vi "IP键盘.vi"(1 "OldNumber":string) -> (0 "NewNumber":string)   [LabVIEW 2016, in "数据传输系统-05.lvlib"]
panel:
  in  "数值":dbl
  in  "Cancel":bool
  in  "OK":bool
  in  "Clear":bool
  in  "BackSpace":bool
  in  "String":string
  in  "Point":bool
  in  "Zero":bool
  in  "Nine":bool
  in  "Eight":bool
  in  "Seven":bool
  in  "Six":bool
  in  "Five":bool
  in  "Four":bool
  in  "Three":bool
  in  "Two":bool
  in  "One":bool
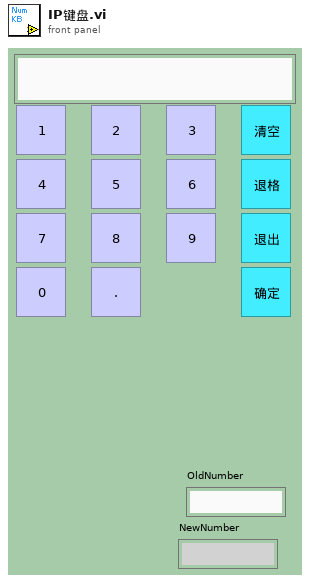
[diagram p1: front panel]
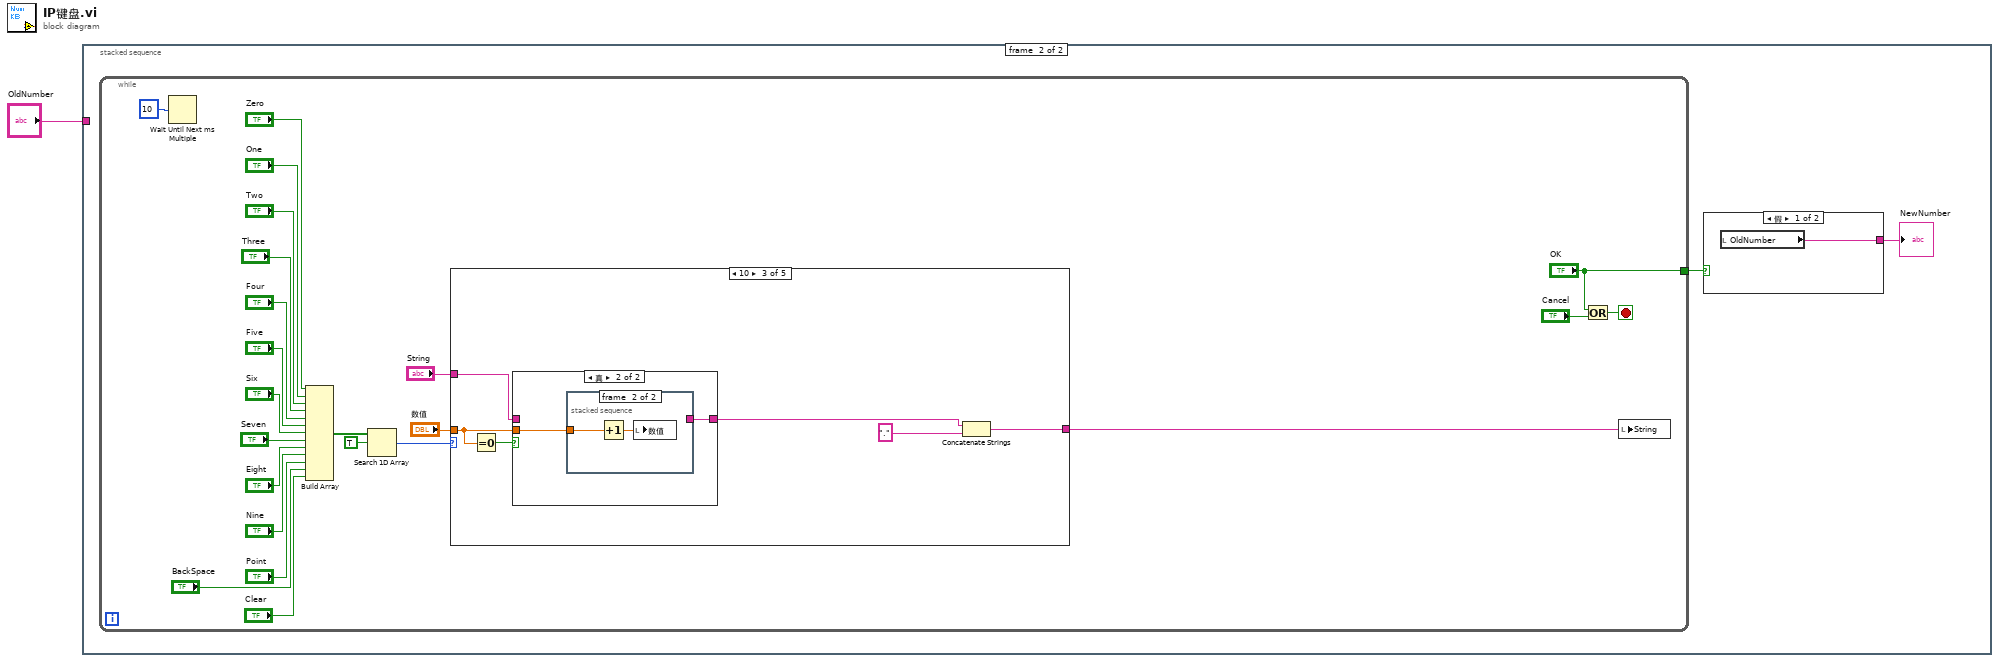
[diagram p0: block diagram]
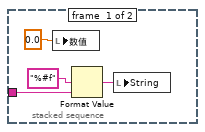
[diagram p2: hidden frame]
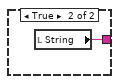
[diagram p3: hidden frame]
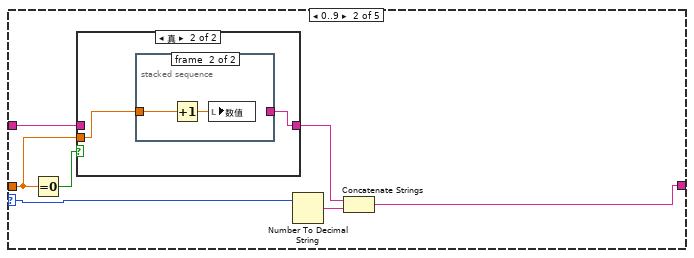
[diagram p5: hidden frame]
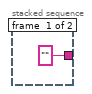
[diagram p7: hidden frame]
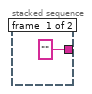
[diagram p9: hidden frame]
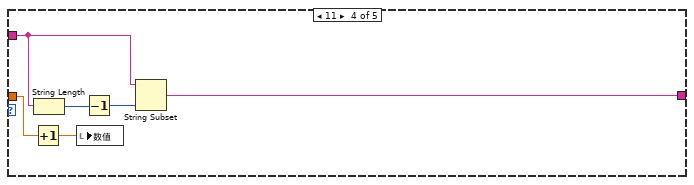
[diagram p10: hidden frame]
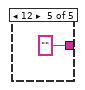
[diagram p11: hidden frame]
diagram:
  n1 = stacked-sequence {
    tunnel: "OldNumber" -> [w2 _]
    frame #0 {
      n2 = local write "数值"(0.0 ("数值")) -> ()
      n3 = Format Value(format string="%#f" ("格式字符串"), value (0)=w2) -> (output string=w3:string)  [unwired: 1 in]
      n4 = local write "String"(w3) -> ()
    }
    frame #1 {
      n5 = while {
        tunnel: ["OK"] -> w7
        stop <- w31 stop-if-true
        n6 = Wait Until Next ms Multiple(millisecond multiple=u32 10) -> ()  [unwired: 1 out]
        n7 = Build Array("Zero", "One", "Two", "Three", "Four", "Five", "Six", "Seven", "Eight", "Nine", "Point", "BackSpace", "Clear") -> (w16:bool[])
        n8 = Search 1D Array(1D array=w16, element=TRUE) -> (index of element=w14:i32)  [unwired: 1 in]
        n9 = case shown="10" w14 {
          selector: w14 -> [_ w40 _ _ _]
          tunnel: "String" -> [w33 w35 w51 w63 _]
          tunnel: [w33 w38 w52 w61 "" ("String")] -> w10
          tunnel: "数值" -> [_ w34 w48 w60 _]
          frame Default {
          }
          frame 0..9 {
            n10 = Equal To 0?(x=w34) -> (x = 0?=w37:bool)
            n11 = case shown="真" w37 {
              tunnel: [w41 w43] -> w36
              tunnel: w34 -> [_ w42]
              tunnel: w35 -> [w41 _]
              frame False {
              }
              frame True {
                n12 = stacked-sequence {
                  tunnel: ["" _] -> w43
                  tunnel: w42 -> [_ w46]
                  frame #0 {
                  }
                  frame #1 {
                    n13 = Increment(x=w46) -> (x+1=w45:dbl)
                    n14 = local write "数值"(w45) -> ()
                  }
                }
              }
            }
            n15 = Number To Decimal String(number=w40) -> (decimal integer string=w39:string)  [unwired: 1 in]
            n16 = Concatenate Strings(w36, w39) -> (w38:string)
          }
          frame 10 {
            n17 = Equal To 0?(x=w48) -> (x = 0?=w50:bool)
            n18 = case shown="真" w50 {
              tunnel: [w53 w55] -> w49
              tunnel: w51 -> [w53 _]
              tunnel: w48 -> [_ w54]
              frame False {
              }
              frame True {
                n19 = stacked-sequence {
                  tunnel: ["" _] -> w55
                  tunnel: w54 -> [_ w57]
                  frame #0 {
                  }
                  frame #1 {
                    n20 = Increment(x=w57) -> (x+1=w58:dbl)
                    n21 = local write "数值"(w58) -> ()
                  }
                }
              }
            }
            n22 = Concatenate Strings(w49, "." ("string")) -> (w52:string)
          }
          frame 11 {
            n23 = Increment(x=w60) -> (x+1=w59:dbl)
            n24 = String Length(string=w63) -> (length=w62:i32)
            n25 = local write "数值"(w59) -> ()
            n26 = Decrement(x=w62) -> (x-1=w64:i32)
            n27 = String Subset(string=w63, length (rest)=w64) -> (substring=w61:string)  [unwired: 1 in]
          }
          frame 12 {
          }
        }
        n28 = Or(x="OK", y="Cancel") -> (x .or. y?=w31:bool)
        n29 = local write "String"(w10) -> ()
      }
      n30 = case shown="假" w7 {
        tunnel: [w8 w9] -> w6
        frame False {
          n31 = local read "OldNumber"() -> (w8:string)
        }
        frame True {
          n32 = local read "String"() -> (w9:string)
        }
      }
      "NewNumber" <- w6
    }
  }
